vi "Ascenseur_Main.vi"() -> ()   [LabVIEW 2026]
panel:
  in  "Descente":bool
  in  "Montée":bool
  out "Vitesse Moteur":dbl
  out "Vitesse sauvegarder":dbl
  in  "Poids Max":dbl
  in  "Vitesse Max":dbl(slide) scale=0.0..10.0
  in  "Alarme":bool
  out "Poids cabine":dbl
  in  "baud rate (9600)":u32=9600
  in  "VISA resource name":refnum<visa-resource-name>
  out "Table Control":string[][](table)
  out "LCD":string
  out "Trames envoyés":string
  out "Trames Recues":string
  out "Dernier étage":dbl
  out "Trajets total":dbl
  out "Statut de connexion":string
  out "Connexion":bool
  out "Capteur IR":bool
  out "EEPROM prête":bool
  out "Cabine en mvt":bool
  out "Mode Manu":bool
  out "Mode Auto":bool
  out "Arrêt urgence":bool
  out "Alarme":bool
  out "Surcharge":bool
  out "Porte Ouverte":bool
  out "Connexion Active":bool
  out "Graphique 2 Poids en fonction du temps":dbl[](graph)
  out "Graphique 1 Position en fonction du temps":dbl[](graph)
  out "Nb trajet":dbl
  out "Direction":string
  out "Etage Actuel":dbl
  in  "Clear TX":bool
  in  "Clear RX":bool
  in  "RAFRAICHIR EEPROM":bool
  in  "ENVOYER CONFIG":bool
  in  "MANU":bool
  in  "AUTO":bool
  in  "Sauvegarder":bool
  in  "Clear":bool
  in  "Stop":bool
  in  "Start":bool
  in  "Déconnecter":bool
  in  "Connecter":bool
  in  "Reset Alarme":bool
  in  "Acquitement":bool
  in  "Arrêt urgence":bool
  in  "Fermeture Porte":bool
  in  "Ouverture Porte":bool
  in  "Etage 2":bool
  in  "Etage  3":bool
  in  "Etage 0":bool
  in  "Etage 1":bool
  # "Projet final du 2ème quadrimestre Système de controle d'ascenseur"
  # "Classe : 2AU"
  # "EL YAZAMI Yassine"
  # "TABICH Mohamed"
  # "Année académique : 2025-2026"
  # "Mode"
  # "Commandes"
  # "ETAT"
  # "INDICATEUR"
  # "Graphiques déroulants"
  # "Appel d'étage"
  # "CONFIG SEUILS"
  # "LCD"
  # "Données EEPROM"
  # "Historique des trajets"
  # "Mode Manuel"
  # "LOG COMMUNICATION"
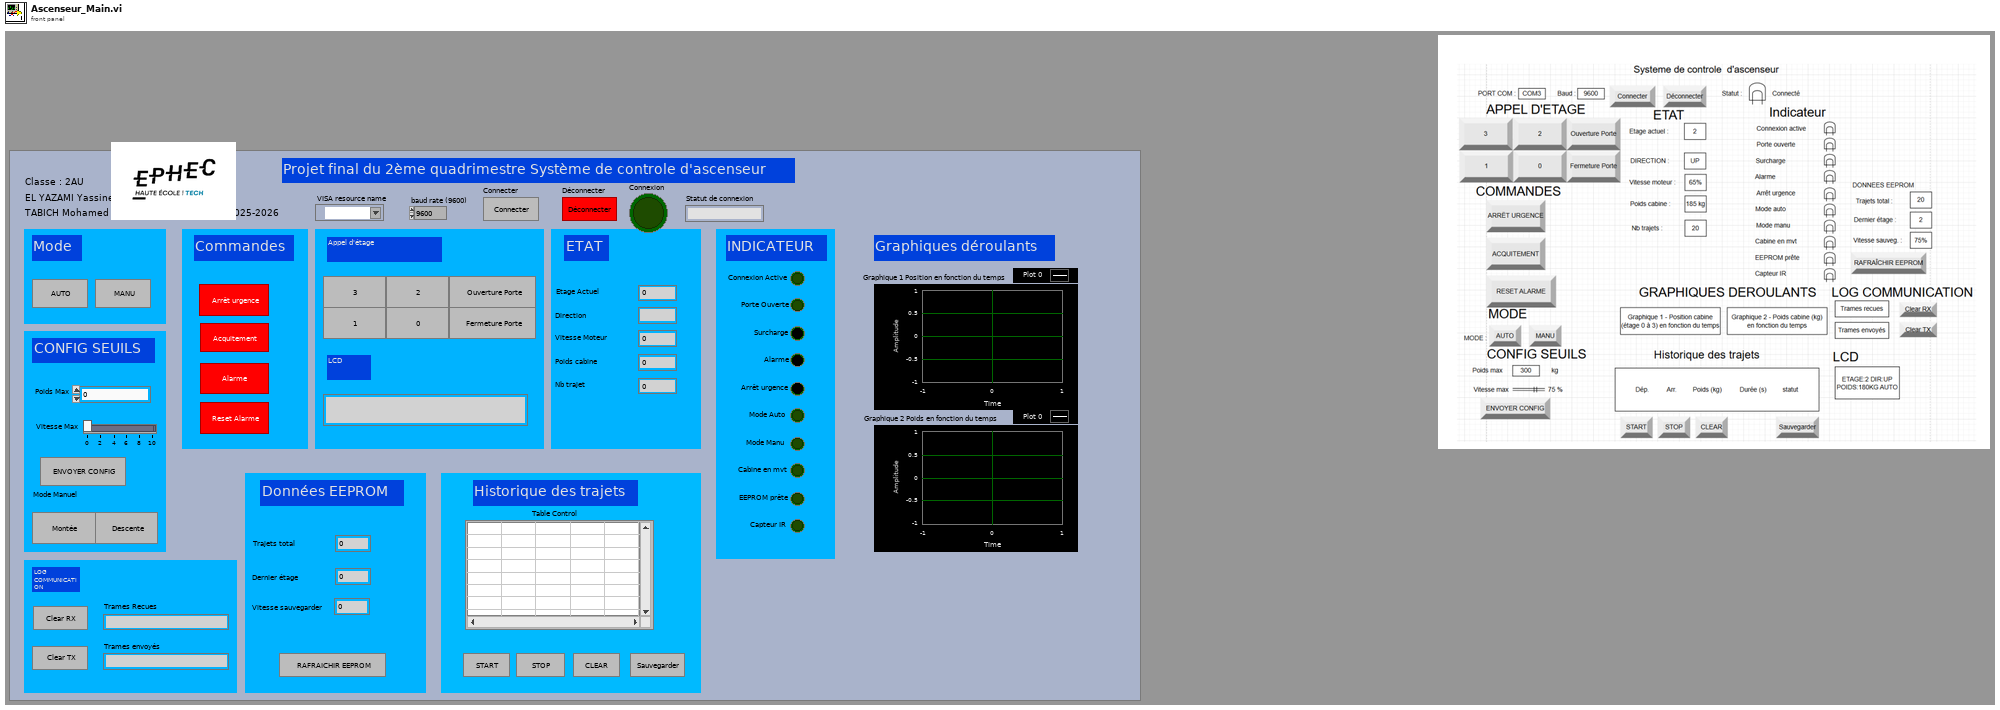
[diagram p1: front panel]
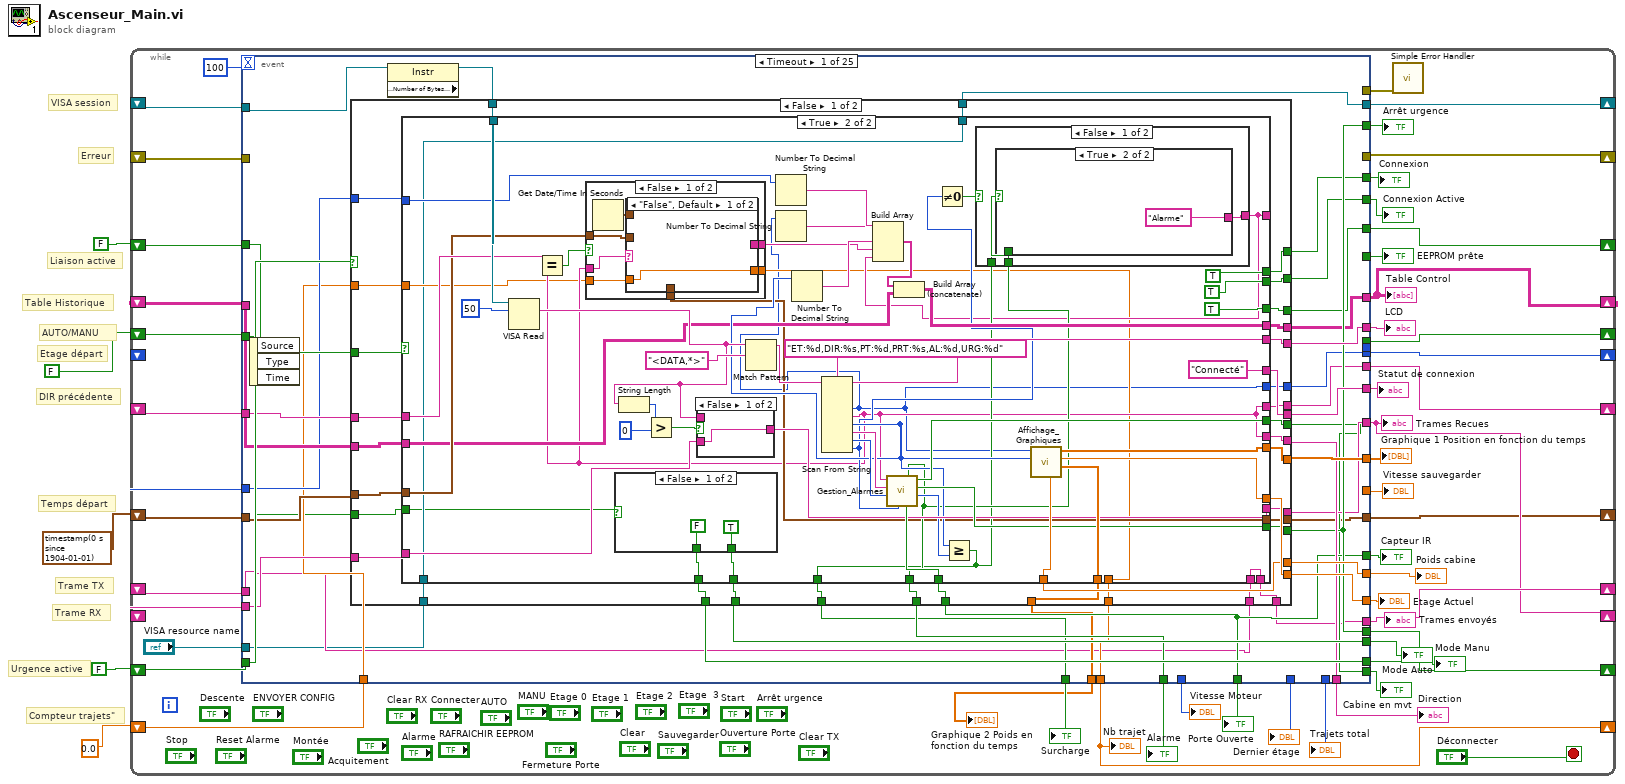
[diagram p0: block diagram]
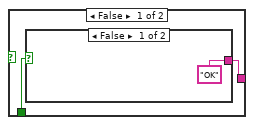
[diagram p3: hidden frame]
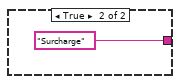
[diagram p4: hidden frame]
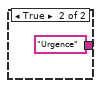
[diagram p5: hidden frame]
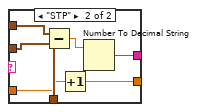
[diagram p6: hidden frame]
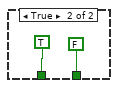
[diagram p9: hidden frame]
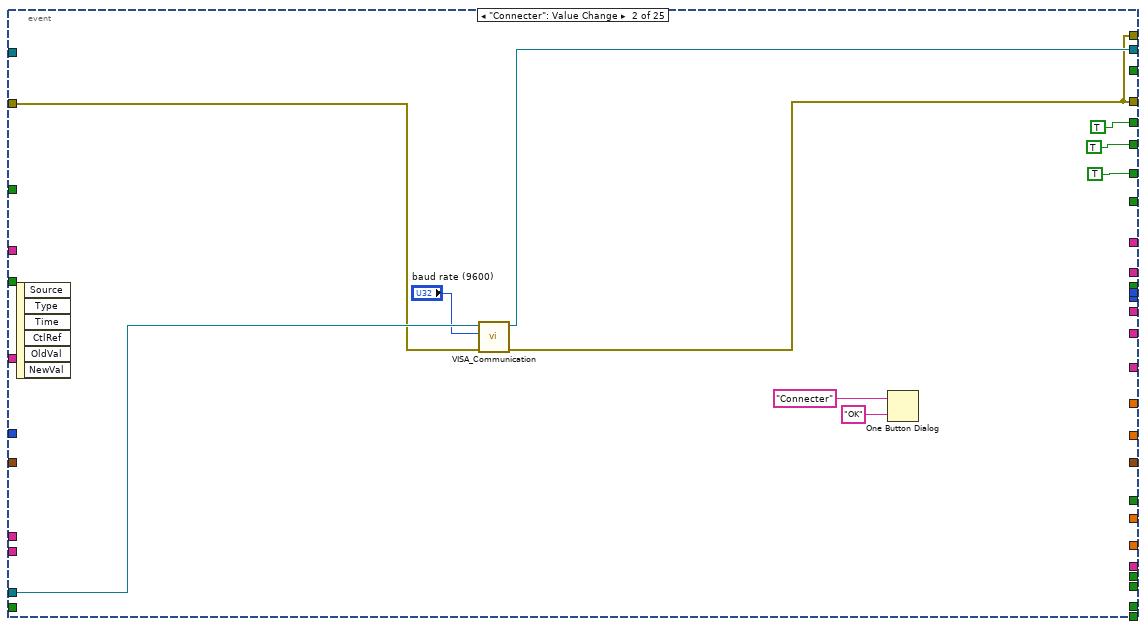
[diagram p11: hidden frame]
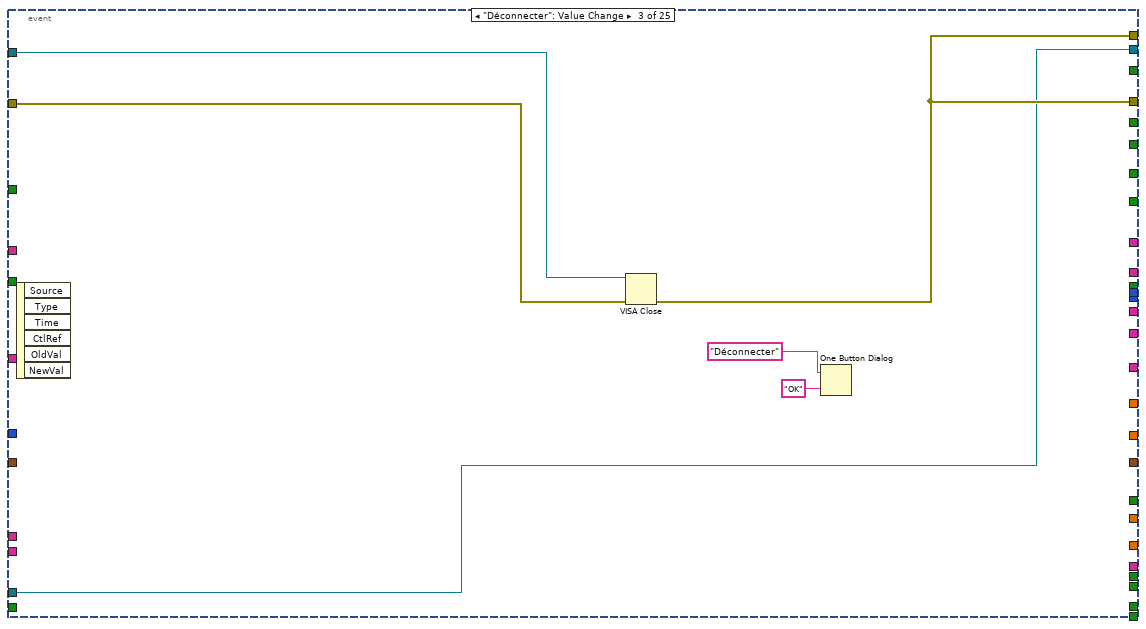
[diagram p12: hidden frame]
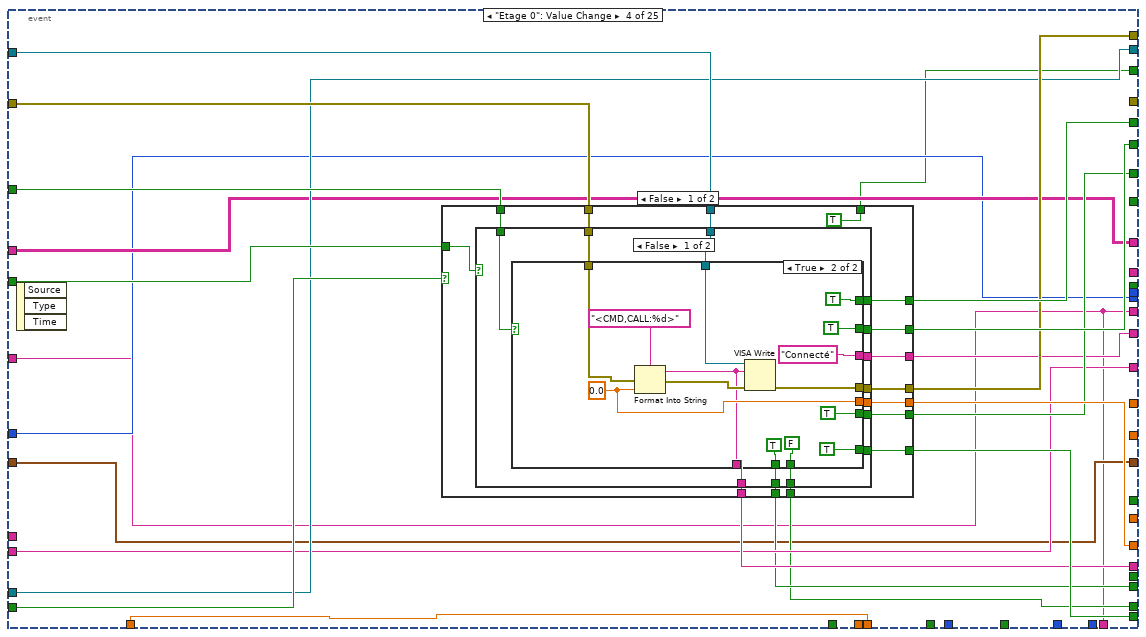
[diagram p13: hidden frame]
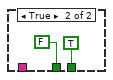
[diagram p15: hidden frame]
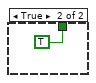
[diagram p16: hidden frame]
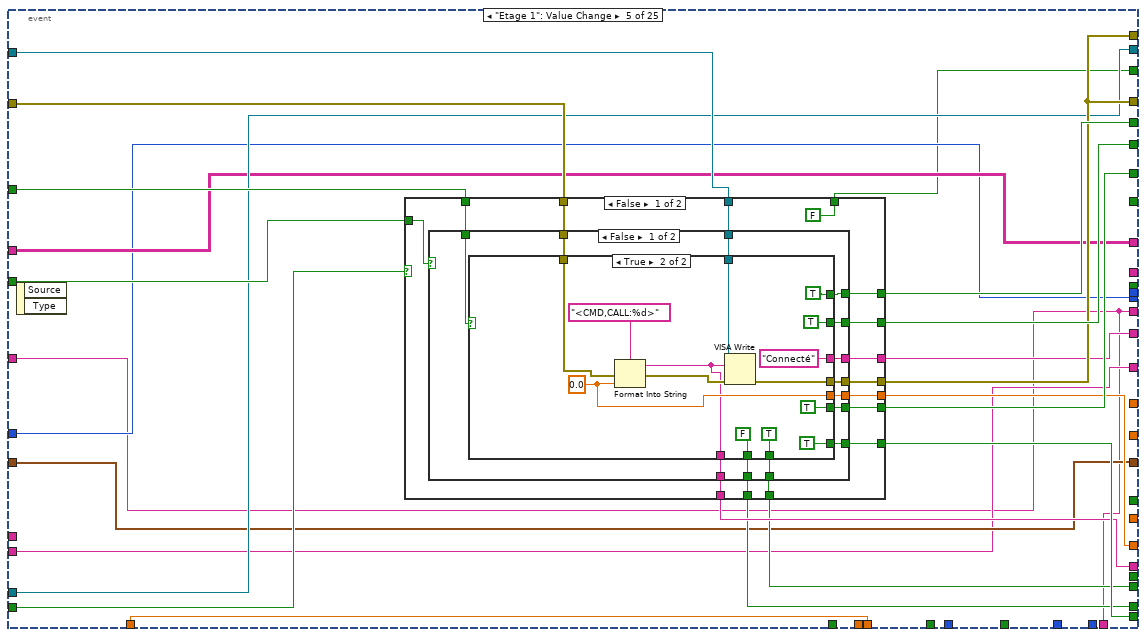
[diagram p17: hidden frame]
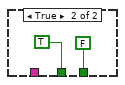
[diagram p19: hidden frame]
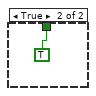
[diagram p20: hidden frame]
diagram:
  # "Compteur trajets\""
  # "Temps départ"
  # "Etage départ"
  # "Table Historique"
  # "DIR précédente"
  # "Trame RX"
  # "Urgence active"
  # "Trame TX"
  # "Erreur"
  # "VISA session"
  # "Liaison active"
  # "AUTO/MANU"
  n1 = while {
    shift-right: [w53] -> _
    shift-left: _ -> [w46]
    shift-right: [w52] -> _
    shift-left: _ -> [w50]
    shift-right: [w48] -> _
    shift-left: FALSE ("Enable Termination\nChar (T)") -> [w49]
    shift-right: [w29] -> _
    shift-left: FALSE ("Mode Auto") -> [w30]
    shift-right: [w28] -> _
    shift-left: _ -> [w45]
    shift-right: [w23] -> _
    shift-left: _ -> [w24]
    shift-right: [w32] -> _
    shift-left: FALSE ("Enable Termination\nChar (T)") -> [w31]
    shift-right: [w17] -> _
    shift-left: _ -> [w18]
    shift-right: [w10] -> _
    shift-left: _ -> [w16]
    shift-right: [w12] -> _
    shift-left: _ -> [w14]
    shift-right: [w11] -> _
    shift-left: timestamp(0 s since 1904-01-01) ("y") -> [w15]
    shift-right: [w7] -> _
    shift-left: 0.0 ("Nb trajet") -> [w9]
    stop <- "Déconnecter" stop-if-true
    n2 = event shown="[0] Timeout" {
      selector: _ -> [_ _ _ _ _ _ _ _ _ _ _ _ _ _ _ _ _ _ _ _ _ _ _ _ _]
      dyn-events: _ -> [_ _ _ _ _ _ _ _ _ _ _ _ _ _ _ _ _ _ _ _ _ _ _ _ _]
      timeout: 100 -> [_ _ _ _ _ _ _ _ _ _ _ _ _ _ _ _ _ _ _ _ _ _ _ _ _]
      tunnel: "VISA resource name" -> [w58 w221 w224 w239 w307 w377 w444 w513 w541 w588 w614 w647 w683 w734 w772 w835 w895 w953 w1006 w1059 w1083 w1115 w1137 w1148 w1175]
      tunnel: [w57 w219 w224 w239 w307 w377 w444 w513 w541 w588 w614 w647 w683 w734 w772 w835 w895 w953 w1006 w1059 w1083 w1115 w1137 w1148 w1175] -> w53
      tunnel: [_ w218 w226 _ w311 w370 w445 w515 w542 w580 w611 w645 w687 w736 w779 w836 w887 w952 w1005 w1056 w1080 w1113 w1134 w1157 w1177] -> w52
      tunnel: [_ w218 w226 w241 w311 w370 w445 w515 w542 w580 w611 w645 w687 w736 w779 w836 w887 w952 w1005 w1056 w1080 w1113 w1134 w1157 w1177] -> w51
      tunnel: w50 -> [_ w217 w225 w246 w309 w386 w439 w516 w544 w589 w618 w649 w693 w735 w782 w846 w897 w951 w1004 w1057 w1081 w1114 w1134 w1158 w1178]
      tunnel: w49 -> [w91 _ _ w249 w316 w380 w450 w511 w539 w585 w615 w646 w695 w739 w775 w834 w900 w955 w1009 w1055 w1076 w1107 w1122 w1155 w1179]
      tunnel: [w72 TRUE ("Enable Termination\nChar (T)") _ w243 w313 w382 w452 w506 w532 w581 w605 w637 w684 w729 w776 w840 w891 _ w1001 w1051 w1077 w1108 w1132 w1159 w1181] -> w48
      tunnel: [w74 TRUE ("Connexion") _ w250 w315 w385 w454 w508 w534 w583 w607 w639 w686 w731 w778 w842 w896 w946 w1003 w1053 w1079 w1110 w1133 w1160 w1183] -> w47
      tunnel: w46 -> [w93 _ w227 w240 w310 w381 w447 w517 w545 w590 w619 w650 w694 w737 w780 w847 w901 w954 w1010 w1058 w1082 _ _ _ _]
      tunnel: w45 -> [w68 _ _ w233 w302 w368 w435 w503 w540 w576 w608 w635 w679 w721 w767 w829 w881 w943 w994 w1048 w1068 _ w1136 w1151 w1172]
      tunnel: [w69 _ _ w233 w302 w368 w435 w503 w543 w576 w608 w635 w679 w721 w767 w829 w881 w943 w994 w1048 w1068 w1112 w1135 w1151 w1172] -> w28
      tunnel: [w73 TRUE ("Connexion Active") _ w244 w314 w384 w453 w507 w533 w582 w606 w638 w685 w730 w777 w841 w892 w949 w1002 w1052 w1078 w1109 w1131 w1156 w1182] -> w44
      tunnel: [w78 _ _ w236 w299 w371 w438 w504 w529 w577 w610 w634 w682 w725 w768 w833 w884 w941 w995 w1050 w1072 w1106 w1126 w1161 w1174] -> w17
      tunnel: [w59 _ _ w237 w305 w375 w442 w512 w536 w587 w616 w640 w692 w726 w769 w837 w888 w945 w998 w1054 w1073 w1105 w1127 w1149 w1180] -> w23
      tunnel: [w88 _ _ w238 w306 w376 w443 w510 w528 w586 w617 w643 w691 w733 w781 w843 w894 w948 w997 w1044 w1074 w1111 w1130 w1154 w1176] -> w43
      tunnel: [w86 _ _ w245 w308 w383 w446 _ _ _ _ _ _ _ _ _ _ _ _ _ _ _ _ _ _] -> w25
      tunnel: [w77 _ _ _ _ _ _ _ _ _ _ _ _ _ _ w839 w889 _ _ _ _ _ _ _ _] -> w42
      tunnel: [w89 _ _ w234 w303 w373 w440 _ _ _ _ _ w689 w727 _ _ w890 w944 w999 _ _ _ _ _ _] -> w41
      tunnel: [w90 _ _ w235 w304 w374 w441 _ _ _ _ _ w690 w728 _ _ _ _ _ _ _ _ _ _ _] -> w40
      tunnel: [w76 _ _ w242 w312 w372 w451 _ _ _ _ _ _ _ _ w838 _ w947 w1000 _ _ _ _ _ _] -> w39
      tunnel: [w80 _ _ w228 w296 w369 w432 w509 w535 w573 w609 _ _ _ _ _ _ _ _ _ _ _ _ _ _] -> w38
      tunnel: [w77 _ _ _ _ _ _ _ _ _ _ _ _ _ _ _ w893 _ _ _ _ _ _ _ _] -> w37
      tunnel: [w82 _ _ _ _ _ _ _ _ w584 w612 _ _ _ _ _ _ _ _ _ _ _ _ _ _] -> w36
      tunnel: [_ _ _ _ _ _ _ _ _ _ _ w642 _ _ _ _ _ _ _ _ _ _ _ _ _] -> w8
      tunnel: [_ _ _ _ _ _ _ _ _ _ _ w648 _ _ _ _ _ _ _ _ _ _ _ _ _] -> w35
      tunnel: [_ _ _ _ _ _ _ _ _ _ _ w644 _ _ w770 _ _ w950 _ _ _ _ _ _ _] -> w34
      tunnel: [w75 _ _ _ _ _ _ _ _ _ w613 _ _ _ _ _ _ _ _ _ _ _ _ _ _] -> w33
      tunnel: [w80 _ _ _ _ _ _ TRUE ("Enable Termination\nChar (T)") w537 _ _ _ _ _ _ _ _ _ _ _ _ _ w1123 w1152 w1173] -> w32
      tunnel: w31 -> [w92 _ _ w247 w318 w378 w448 _ w538 _ _ _ w696 w738 w774 w844 w898 w957 w1007 _ w1075 _ w1123 w1152 w1173]
      tunnel: w30 -> [w56 _ _ w248 w317 w379 w449 _ _ _ _ _ _ _ w773 w845 w899 w956 w1008 _ _ _ _ w1153 _]
      tunnel: [_ _ _ _ _ _ _ _ _ _ _ _ w688 w732 _ _ _ _ _ _ _ _ _ w1153 _] -> w29
      tunnel: [_ _ _ _ _ _ _ _ _ _ _ _ _ _ w771 _ _ _ _ _ _ _ _ _ _] -> w27
      tunnel: [_ _ _ _ _ _ _ _ _ _ _ w641 _ _ _ _ _ _ _ _ _ _ _ _ _] -> w26
      tunnel: w24 -> [w60 _ _ _ _ _ _ _ _ _ _ _ _ _ _ _ _ _ _ _ _ w1105 w1127 w1149 _]
      tunnel: [w87 _ _ _ _ _ _ _ _ _ _ _ _ _ _ _ _ _ _ _ _ _ _ _ _] -> w22
      tunnel: [w85 _ _ _ _ _ _ _ _ _ _ _ _ _ _ _ _ _ _ _ _ _ _ _ _] -> w21
      tunnel: [w84 _ _ _ _ _ _ _ _ _ _ _ _ _ _ _ _ _ _ _ _ _ _ _ _] -> w20
      tunnel: [w83 _ _ w229 w297 w364 w433 _ _ w574 w601 _ _ _ _ _ _ w939 w991 w1044 _ _ w1124 _ _] -> w19
      tunnel: w18 -> [w79 _ _ w236 w299 w371 w438 w504 w529 w577 w610 w634 w682 w725 w768 w833 w884 w941 w995 w1050 w1072 w1106 w1126 _ w1174]
      tunnel: w16 -> [w71 _ _ w229 w297 w364 w433 w505 w530 w574 w601 w636 w680 w723 w766 w828 w885 w939 w991 w1049 w1069 w1103 w1124 w1150 w1170]
      tunnel: w15 -> [w70 _ _ w231 w300 w366 w436 w500 _ w578 w603 w631 w678 w722 w765 w831 w882 w938 w992 w1045 w1071 w1102 w1129 w1146 w1171]
      tunnel: w14 -> [w67 _ _ w232 w301 w367 w434 w501 w527 w579 w604 w632 w681 w720 w763 w830 w886 w942 w993 w1046 w1070 w1104 w1125 w1147 w1168]
      tunnel: [w66 _ _ _ _ _ _ _ _ _ _ _ _ _ _ _ _ _ _ _ _ _ _ _ _] -> w13
      tunnel: [w65 _ _ w232 w301 w367 w434 w501 w527 w579 w604 w632 w681 w720 w763 w830 w886 w942 w993 w1046 w1070 w1104 w1125 w1147 _] -> w12
      tunnel: [w64 _ _ w231 w300 w366 w436 w500 _ w578 w603 w631 w678 w722 w765 w831 w882 w938 w992 w1045 w1071 w1102 w1129 w1146 w1171] -> w11
      tunnel: [w63 _ _ w229 w297 w364 w433 w505 w530 w574 w601 w636 w680 w723 w766 w828 w885 w939 w991 w1049 w1069 w1103 w1124 w1150 w1170] -> w10
      tunnel: w9 -> [w62 _ _ w230 w298 w365 w437 w502 w531 w575 w602 w633 w677 w724 w764 w832 w883 w940 w996 w1047 _ w1101 w1128 w1145 w1169]
      tunnel: [w61 _ _ w230 w298 w365 w437 w502 w531 w575 w602 w633 w677 w724 w764 w832 w883 w940 w996 w1047 _ w1101 w1128 w1145 w1169] -> w7
      tunnel: [_ _ _ _ _ _ _ _ _ _ _ _ _ _ _ _ _ _ _ _ _ _ _ _ w1168] -> _
      event Timeout {
        n3 = event-data() -> ()  [unwired: 1 in, 3 out]
        n4 = property class="Instr" props=["Serial Settings:Number of Bytes at Serial Port"](reference=w93) -> (reference out=w81:refnum<visa-resource-name>)  [unwired: 1 in, 2 out]
        n5 = case shown="False" w92 {
          tunnel: w91 -> [w129 _]
          tunnel: [w128 _] -> w90
          tunnel: [w127 _] -> w89
          tunnel: [w126 _] -> w88
          tunnel: [w125 _] -> w87
          tunnel: [w124 _] -> w86
          tunnel: [w123 _] -> w85
          tunnel: [w122 _] -> w66
          tunnel: [w121 _] -> w84
          tunnel: [w120 _] -> w83
          tunnel: [w119 _] -> w82
          tunnel: [w118 _] -> w77
          tunnel: w81 -> [w117 _]
          tunnel: [w116 _] -> w80
          tunnel: w79 -> [w115 _]
          tunnel: [w114 _] -> w78
          tunnel: [w113 _] -> w76
          tunnel: [w112 _] -> w75
          tunnel: [w111 _] -> w74
          tunnel: [w110 _] -> w73
          tunnel: [w109 _] -> w72
          tunnel: w71 -> [w108 _]
          tunnel: w70 -> [w107 _]
          tunnel: [w106 _] -> w69
          tunnel: w68 -> [w105 _]
          tunnel: w67 -> [w104 _]
          tunnel: [w103 _] -> w65
          tunnel: [w102 _] -> w64
          tunnel: [w101 _] -> w63
          tunnel: w62 -> [w100 _]
          tunnel: [w99 _] -> w61
          tunnel: w60 -> [w98 _]
          tunnel: [w97 _] -> w59
          tunnel: w58 -> [w96 _]
          tunnel: [w95 _] -> w57
          tunnel: w56 -> [w94 _]
          frame False {
            n6 = case shown="True" w129 {
              tunnel: [_ w136] -> w120
              tunnel: [_ w177] -> w118
              tunnel: [_ w140] -> w119
              tunnel: [_ w175] -> w121
              tunnel: [_ w174] -> w125
              tunnel: [_ w173] -> w124
              tunnel: [_ w172] -> w123
              tunnel: [_ w171] -> w122
              tunnel: [_ "Connecté" ("Statut de connexion")] -> w126
              tunnel: [_ w169] -> w128
              tunnel: [_ w168] -> w127
              tunnel: w117 -> [_ w167]
              tunnel: [_ w166] -> w116
              tunnel: w115 -> [_ w160]
              tunnel: [_ w161] -> w114
              tunnel: [_ w159] -> w113
              tunnel: [_ w139] -> w112
              tunnel: [_ TRUE ("Connexion")] -> w111
              tunnel: [_ TRUE ("Connexion Active")] -> w110
              tunnel: [_ TRUE ("Enable Termination\nChar (T)")] -> w109
              tunnel: w108 -> [_ w153]
              tunnel: w107 -> [_ w152]
              tunnel: [_ w151] -> w106
              tunnel: w105 -> [_ w144]
              tunnel: w104 -> [_ w150]
              tunnel: [_ w138] -> _
              tunnel: [_ w130] -> w103
              tunnel: [_ w137] -> w102
              tunnel: [_ w136] -> w101
              tunnel: w100 -> [_ w135]
              tunnel: [_ w134] -> w99
              tunnel: w98 -> [_ w133]
              tunnel: [_ w133] -> w97
              tunnel: [_ w132] -> w95
              tunnel: w96 -> [_ w132]
              tunnel: w94 -> [_ w131]
              frame False {
              }
              frame True {
                n7 = VISA Read(VISA resource name=w167, byte count=u32 50) -> (read buffer=w162:string)  [unwired: 1 in, 3 out]
                n8 = case shown="False" w131 {
                  tunnel: [TRUE ("Mode Auto") FALSE ("Mode Auto")] -> w169
                  tunnel: [FALSE ("Mode Manu") TRUE ("Mode Manu")] -> w168
                  frame False {
                  }
                  frame True {
                  }
                }
                n9 = String Length(string=w162) -> (length=w164:i32)
                n10 = Greater?(x=w164, y=0 ("length")) -> (0:w163:bool)
                n11 = case shown="False" w163 {
                  tunnel: [w206 w207] -> w161
                  tunnel: w162 -> [_ w207]
                  tunnel: w160 -> [w206 _]
                  frame False {
                  }
                  frame True {
                  }
                }
                n12 = Match Pattern(string=w162, regular expression="<DATA,*>") -> (after substring=w180:string)  [unwired: 1 in, 3 out]
                n13 = Number To Decimal String(number=w150) -> (decimal integer string=w148:string)  [unwired: 1 in]
                n14 = Scan From String(format string="ET:%d,DIR:%s,PT:%d,PRT:%s,AL:%d,URG:%d", input string=w180) -> (remaining string=w175:string, output 1=w130:i32, output 2=w136:string, output 3=w149:i32, output 4=w178:string, output 5=w176:i32, output 6=w141:i32)  [unwired: 8 in, 2 out]
                n15 = Equal?(x=w153, y=w136) -> (x = y?=w154:bool)
                n16 = case shown="False" w154 {
                  tunnel: w136 -> [w198 _]
                  tunnel: w152 -> [w196 _]
                  tunnel: [w195 _] -> w145
                  tunnel: [w194 _] -> w137
                  tunnel: w135 -> [w193 _]
                  tunnel: [w192 _] -> w134
                  frame False {
                    n17 = Get Date/Time In Seconds() -> (seconds since 1Jan1904=w197:timestamp)
                    n18 = case shown="\"False\", Default" w198 {
                      tunnel: w197 -> [_ w205]
                      tunnel: w196 -> [_ w202]
                      tunnel: [_ w203] -> w195
                      tunnel: [_ w202] -> w194
                      tunnel: w193 -> [w199 w201]
                      tunnel: [w199 w200] -> w192
                      frame "False", Default {
                      }
                      frame "STP" {
                        n19 = Subtract(x=w205, y=w202) -> (x-y=w204:dbl)
                        n20 = Increment(x=w201) -> (x+1=w200:dbl)
                        n21 = Number To Decimal String(number=w204) -> (decimal integer string=w203:string)  [unwired: 1 in]
                      }
                    }
                  }
                  frame True {
                  }
                }
                n22 = Number To Decimal String(number=w130) -> (decimal integer string=w147:string)  [unwired: 1 in]
                n23 = Number To Decimal String(number=w149) -> (decimal integer string=w146:string)  [unwired: 1 in]
                n24 = call "Gestion_Alarmes.vi"("Numeric"=w141, "Numeric 2"=w176, "String 2"=w178, "String"=w136) -> ("y"=w158:i32, "Boolean 3"=w166:bool, "Boolean 2"=w159:bool, "Boolean 4"=w177:bool, "Boolean"=w140:bool)  [unwired: 3 in]
                n25 = Not Equal To 0?(x=w141) -> (x != 0?=w142:bool)
                n26 = Greater Or Equal?(x=w149, y=w158) -> (x >= y?=w139:bool)
                n27 = case shown="False" w142 {
                  tunnel: w140 -> [w185 _]
                  tunnel: w139 -> [w184 _]
                  tunnel: [w183 "Urgence"] -> w138
                  frame False {
                    n28 = case shown="True" w185 {
                      tunnel: w184 -> [w187 _]
                      tunnel: [w186 "Alarme"] -> w183
                      frame False {
                        n29 = case shown="False" w187 {
                          tunnel: ["OK" "Surcharge"] -> w186
                          frame False {
                          }
                          frame True {
                          }
                        }
                      }
                      frame True {
                      }
                    }
                  }
                  frame True {
                  }
                }
                n30 = Build Array(w148, w147, w146, w145, w138) -> (w143:string[])
                n31 = Build Array (concatenate)(w143, w144) -> (w151:string[][])
                n32 = call "Affichage_Graphiques.vi"("Poids"=w149, "Position"=w130) -> ("Graphique 2 Poids en fonction du temps"=w171:dbl[], "Etage Actuel"=w173:dbl, "Graphique 1 Position en fonction du temps"=w174:dbl[], "Poids cabine"=w172:dbl)  [unwired: 6 in]
              }
            }
          }
          frame True {
          }
        }
      }
      event "Connecter": Value Change {
        n33 = event-data() -> ()  [unwired: 1 in, 6 out]
        n34 = call "VISA_Communication.vi"("error in (no error)"=w217, "baud rate (9600)"="baud rate (9600)", "VISA Refnum in"=w221) -> ("error out"=w218:errorcluster, "VISA Refnum out"=w219:refnum<visa-resource-name>)  [unwired: 7 in]
        n35 = One Button Dialog(message="Connecter", button name ("OK")="OK") -> ()  [unwired: 1 out]
      }
      event "Déconnecter": Value Change {
        n36 = event-data() -> ()  [unwired: 1 in, 6 out]
        n37 = VISA Close(VISA resource name=w227, error in (no error)=w225) -> (error out=w226:errorcluster)
        n38 = One Button Dialog(message="Déconnecter", button name ("OK")="OK") -> ()  [unwired: 1 out]
      }
      event "Etage 0": Value Change {
        n39 = event-data() -> ()  [unwired: 1 in, 3 out]
        n40 = case shown="False" w247 {
          tunnel: [w265 _] -> w250
          tunnel: w249 -> [w264 _]
          tunnel: w248 -> [w263 _]
          tunnel: w246 -> [w262 _]
          tunnel: [w261 _] -> w245
          tunnel: [w260 _] -> w244
          tunnel: [w259 _] -> w243
          tunnel: [w258 _] -> w242
          tunnel: [w257 _] -> w241
          tunnel: w240 -> [w256 _]
          tunnel: [w255 _] -> w238
          tunnel: [w254 _] -> w237
          tunnel: [w253 _] -> w235
          tunnel: [w252 _] -> w234
          tunnel: [TRUE ("Connexion") TRUE ("Connexion")] -> w228
          frame False {
            n41 = case shown="False" w263 {
              tunnel: [w278 _] -> w265
              tunnel: w264 -> [w277 _]
              tunnel: w262 -> [w276 _]
              tunnel: [w275 _] -> w261
              tunnel: [w274 _] -> w260
              tunnel: [w273 _] -> w259
              tunnel: [w272 _] -> w258
              tunnel: [w271 _] -> w257
              tunnel: w256 -> [w270 _]
              tunnel: [w269 _] -> w255
              tunnel: [w268 _] -> w254
              tunnel: [w267 FALSE ("Mode Auto")] -> w253
              tunnel: [w266 TRUE ("Mode Manu")] -> w252
              frame False {
                n42 = case shown="True" w277 {
                  tunnel: [_ w291] -> w271
                  tunnel: [_ TRUE ("Enable Termination\nChar (T)")] -> w273
                  tunnel: [_ TRUE ("Connexion")] -> w278
                  tunnel: [_ w287] -> w275
                  tunnel: [_ TRUE ("Cabine en mvt")] -> w272
                  tunnel: w276 -> [_ w285]
                  tunnel: [_ TRUE ("Connexion Active")] -> w274
                  tunnel: w270 -> [_ w283]
                  tunnel: [_ "Connecté" ("Statut de connexion")] -> w269
                  tunnel: [_ w281] -> w268
                  tunnel: [_ TRUE ("Mode Auto")] -> w267
                  tunnel: [_ FALSE ("Mode Manu")] -> w266
                  frame False {
                  }
                  frame True {
                    w287 = 0.0 ("input 1")
                    n43 = Format Into String(format string="<CMD,CALL:%d>", error in=w285, w287) -> (resulting string=w281:string, error out=w288:errorcluster)  [unwired: 1 in]
                    n44 = VISA Write(VISA resource name=w283, write buffer=w281, error in (no error)=w288) -> (error out=w291:errorcluster)  [unwired: 2 out]
                  }
                }
              }
              frame True {
              }
            }
          }
          frame True {
          }
        }
      }
      event "Etage 1": Value Change {
        n45 = event-data() -> ()  [unwired: 1 in, 2 out]
        n46 = case shown="False" w318 {
          tunnel: [w333 _] -> w315
          tunnel: [w332 _] -> w308
          tunnel: [w331 _] -> w314
          tunnel: [w330 _] -> w313
          tunnel: [w329 _] -> w312
          tunnel: w317 -> [w328 _]
          tunnel: w316 -> [w327 _]
          tunnel: [w326 _] -> w311
          tunnel: w310 -> [w325 _]
          tunnel: w309 -> [w324 _]
          tunnel: [w323 _] -> w306
          tunnel: [w322 _] -> w305
          tunnel: [w321 _] -> w304
          tunnel: [w320 _] -> w303
          tunnel: [FALSE ("Connexion") TRUE ("Connexion")] -> w296
          frame False {
            n47 = case shown="False" w328 {
              tunnel: [w346 _] -> w333
              tunnel: [w345 _] -> w332
              tunnel: [w344 _] -> w331
              tunnel: [w343 _] -> w330
              tunnel: [w342 _] -> w329
              tunnel: w327 -> [w341 _]
              tunnel: [w340 _] -> w326
              tunnel: w325 -> [w339 _]
              tunnel: w324 -> [w338 _]
              tunnel: [w337 _] -> w323
              tunnel: [w336 _] -> w322
              tunnel: [w335 FALSE ("Mode Auto")] -> w321
              tunnel: [w334 TRUE ("Mode Manu")] -> w320
              frame False {
                n48 = case shown="True" w341 {
                  tunnel: [_ w359] -> w340
                  tunnel: [_ TRUE ("Enable Termination\nChar (T)")] -> w343
                  tunnel: [_ TRUE ("Connexion")] -> w346
                  tunnel: [_ w355] -> w345
                  tunnel: [_ TRUE ("Cabine en mvt")] -> w342
                  tunnel: [_ TRUE ("Connexion Active")] -> w344
                  tunnel: w339 -> [_ w352]
                  tunnel: w338 -> [_ w351]
                  tunnel: [_ "Connecté" ("Statut de connexion")] -> w337
                  tunnel: [_ w349] -> w336
                  tunnel: [_ TRUE ("Mode Auto")] -> w335
                  tunnel: [_ FALSE ("Mode Manu")] -> w334
                  frame False {
                  }
                  frame True {
                    w355 = 0.0 ("input 1")
                    n49 = Format Into String(format string="<CMD,CALL:%d>", error in=w351, w355) -> (resulting string=w349:string, error out=w356:errorcluster)  [unwired: 1 in]
                    n50 = VISA Write(VISA resource name=w352, write buffer=w349, error in (no error)=w356) -> (error out=w359:errorcluster)  [unwired: 2 out]
                  }
                }
              }
              frame True {
              }
            }
          }
          frame True {
          }
        }
      }
      event "Etage 2": Value Change {
        n51 = event-data() -> ()  [unwired: 1 in, 3 out]
        n52 = case shown="False" w378 {
          tunnel: [w401 _] -> w385
          tunnel: [w400 _] -> w383
          tunnel: [w399 _] -> w384
          tunnel: [w398 _] -> w382
          tunnel: [w397 _] -> w372
          tunnel: [w396 _] -> w370
          tunnel: w386 -> [w395 _]
          tunnel: w381 -> [w394 _]
          tunnel: w380 -> [w393 _]
          tunnel: w379 -> [w392 _]
          tunnel: [w391 _] -> w376
          tunnel: [w390 _] -> w375
          tunnel: [w389 _] -> w374
          tunnel: [w388 _] -> w373
          tunnel: [FALSE ("Arrêt urgence") TRUE ("Arrêt urgence")] -> w369
          frame False {
            n53 = case shown="False" w392 {
              tunnel: [w414 _] -> w401
              tunnel: [w413 _] -> w400
              tunnel: [w412 _] -> w399
              tunnel: [w411 _] -> w398
              tunnel: [w410 _] -> w397
              tunnel: [w409 _] -> w396
              tunnel: w395 -> [w408 _]
              tunnel: w394 -> [w407 _]
              tunnel: w393 -> [w406 _]
              tunnel: [w405 _] -> w391
              tunnel: [w404 _] -> w390
              tunnel: [w403 FALSE ("Mode Auto")] -> w389
              tunnel: [w402 TRUE ("Mode Manu")] -> w388
              frame False {
                n54 = case shown="True" w406 {
                  tunnel: [_ w427] -> w409
                  tunnel: [_ TRUE ("Enable Termination\nChar (T)")] -> w411
                  tunnel: [_ TRUE ("Connexion")] -> w414
                  tunnel: [_ w423] -> w413
                  tunnel: [_ TRUE ("Cabine en mvt")] -> w410
                  tunnel: [_ TRUE ("Connexion Active")] -> w412
                  tunnel: w408 -> [_ w420]
                  tunnel: w407 -> [_ w419]
                  tunnel: [_ "Connecté" ("Statut de connexion")] -> w405
                  tunnel: [_ w417] -> w404
                  tunnel: [_ TRUE ("Mode Auto")] -> w403
                  tunnel: [_ FALSE ("Mode Manu")] -> w402
                  frame False {
                  }
                  frame True {
                    w423 = 0.0 ("input 1")
                    n55 = Format Into String(format string="<CMD,CALL:%d>", error in=w420, w423) -> (resulting string=w417:string, error out=w424:errorcluster)  [unwired: 1 in]
                    n56 = VISA Write(VISA resource name=w419, write buffer=w417, error in (no error)=w424) -> (error out=w427:errorcluster)  [unwired: 2 out]
                  }
                }
              }
              frame True {
              }
            }
          }
          frame True {
          }
        }
      }
      event "Etage  3": Value Change {
        n57 = event-data() -> ()  [unwired: 1 in, 3 out]
        n58 = case shown="False" w448 {
          tunnel: [w469 _] -> w454
          tunnel: [w468 _] -> w446
          tunnel: [w467 _] -> w453
          tunnel: [w466 _] -> w452
          tunnel: [w465 _] -> w451
          tunnel: [w464 _] -> w445
          tunnel: w450 -> [w463 _]
          tunnel: w449 -> [w462 _]
          tunnel: w447 -> [w461 _]
          tunnel: [w460 _] -> w443
          tunnel: [w459 _] -> w442
          tunnel: [w458 _] -> w441
          tunnel: [w457 _] -> w440
          tunnel: w439 -> [w456 _]
          tunnel: [FALSE ("Arrêt urgence") TRUE ("Arrêt urgence")] -> w432
          frame False {
            n59 = case shown="False" w462 {
              tunnel: [w482 _] -> w469
              tunnel: [w481 _] -> w468
              tunnel: [w480 _] -> w467
              tunnel: [w479 _] -> w466
              tunnel: [w478 _] -> w465
              tunnel: [w477 _] -> w464
              tunnel: w463 -> [w476 _]
              tunnel: w461 -> [w475 _]
              tunnel: [w474 _] -> w460
              tunnel: [w473 _] -> w459
              tunnel: [w472 FALSE ("Mode Auto")] -> w458
              tunnel: [w471 TRUE ("Mode Manu")] -> w457
              tunnel: w456 -> [w470 _]
              frame False {
                n60 = case shown="True" w476 {
                  tunnel: [_ w495] -> w477
                  tunnel: [_ TRUE ("Enable Termination\nChar (T)")] -> w479
                  tunnel: [_ TRUE ("Connexion")] -> w482
                  tunnel: [_ w491] -> w481
                  tunnel: [_ TRUE ("Cabine en mvt")] -> w478
                  tunnel: [_ TRUE ("Connexion Active")] -> w480
                  tunnel: w475 -> [_ w488]
                  tunnel: [_ "Connecté" ("Statut de connexion")] -> w474
                  tunnel: [_ w486] -> w473
                  tunnel: [_ TRUE ("Mode Auto")] -> w472
                  tunnel: [_ FALSE ("Mode Manu")] -> w471
                  tunnel: w470 -> [_ w483]
                  frame False {
                  }
                  frame True {
                    w491 = 0.0 ("input 1")
                    n61 = Format Into String(format string="<CMD,CALL:%d>", error in=w483, w491) -> (resulting string=w486:string, error out=w492:errorcluster)  [unwired: 1 in]
                    n62 = VISA Write(VISA resource name=w488, write buffer=w486, error in (no error)=w492) -> (error out=w495:errorcluster)  [unwired: 2 out]
                  }
                }
              }
              frame True {
              }
            }
          }
          frame True {
          }
        }
      }
      event "Arrêt urgence": Value Change {
        n63 = event-data() -> ()  [unwired: 1 in, 3 out]
        n64 = case shown="True" w511 {
          tunnel: w517 -> [_ w526]
          tunnel: w516 -> [_ w525]
          tunnel: [_ w524] -> w515
          tunnel: [_ w523] -> w512
          tunnel: [_ "URGENCE DÉCLENCHÉE" ("Statut de connexion")] -> w510
          tunnel: [_ TRUE ("Arrêt urgence")] -> w509
          tunnel: [_ TRUE ("Connexion")] -> w508
          tunnel: [_ TRUE ("Connexion Active")] -> w507
          tunnel: [_ TRUE ("Enable Termination\nChar (T)")] -> w506
          frame False {
          }
          frame True {
            w523 = "<CMD,STOP>"
            n65 = VISA Write(VISA resource name=w526, write buffer=w523, error in (no error)=w525) -> (error out=w524:errorcluster)  [unwired: 2 out]
          }
        }
      }
      event "Acquitement": Value Change {
        n66 = event-data() -> ()  [unwired: 1 in, 3 out]
        n67 = case shown="True" w538 {
          tunnel: w545 -> [_ w558]
          tunnel: w544 -> [_ w557]
          tunnel: [_ w556] -> w543
          tunnel: [_ w555] -> w542
          tunnel: w540 -> [_ w554]
          tunnel: w539 -> [_ w553]
          tunnel: [_ w552] -> w537
          tunnel: [_ w551] -> w536
          tunnel: [_ w550] -> w535
          tunnel: [_ w549] -> w534
          tunnel: [_ w548] -> w533
          tunnel: [_ w547] -> w532
          tunnel: [_ w546] -> w528
          frame False {
          }
          frame True {
            n68 = case shown="True" w553 {
              tunnel: w558 -> [_ w572]
              tunnel: w557 -> [_ w571]
              tunnel: [_ w568] -> w556
              tunnel: [_ w567] -> w555
              tunnel: w554 -> [_ w565]
              tunnel: [_ FALSE ("Enable Termination\nChar (T)")] -> w552
              tunnel: [_ w564] -> w551
              tunnel: [_ FALSE ("Arrêt urgence")] -> w550
              tunnel: [_ TRUE ("Connexion")] -> w549
              tunnel: [_ TRUE ("Connexion Active")] -> w548
              tunnel: [_ TRUE ("Enable Termination\nChar (T)")] -> w547
              tunnel: [_ "Système réinitialisé" ("Statut de connexion")] -> w546
              frame False {
              }
              frame True {
                w564 = "<CMD,ACK> "
                n69 = Build Array("TX: <CMD,ACK> " ("Statut de connexion")) -> (w569:string[])
                n70 = VISA Write(VISA resource name=w572, write buffer=w564, error in (no error)=w571) -> (error out=w567:errorcluster)  [unwired: 2 out]
                n71 = Build Array (concatenate)(w569, w565) -> (w568:string[][])
              }
            }
          }
        }
      }
      event "Alarme": Value Change {
        n72 = event-data() -> ()  [unwired: 1 in, 3 out]
        n73 = case shown="True" w585 {
          tunnel: w590 -> [_ w600]
          tunnel: w589 -> [_ w599]
          tunnel: [_ w596] -> w580
          tunnel: [_ w598] -> w587
          tunnel: [_ "Alarme déclenchée " ("Statut de connexion")] -> w586
          tunnel: [_ TRUE] -> w584
          tunnel: [_ TRUE ("Connexion")] -> w583
          tunnel: [_ TRUE ("Connexion Active")] -> w582
          tunnel: [_ TRUE ("Enable Termination\nChar (T)")] -> w581
          tunnel: [_ FALSE ("Arrêt urgence")] -> w573
          frame False {
          }
          frame True {
            w598 = "<CMD,AL:ON> "
            n74 = VISA Write(VISA resource name=w600, write buffer=w598, error in (no error)=w599) -> (error out=w596:errorcluster)  [unwired: 2 out]
          }
        }
      }
      event "Reset Alarme": Value Change {
        n75 = event-data() -> ()  [unwired: 1 in, 3 out]
        n76 = case shown="True" w615 {
          tunnel: w619 -> [_ w630]
          tunnel: w618 -> [_ w629]
          tunnel: [_ w628] -> w611
          tunnel: [_ "Alarmes réinitialisées " ("Statut de connexion")] -> w617
          tunnel: [_ w626] -> w616
          tunnel: [_ FALSE ("Surcharge")] -> w613
          tunnel: [_ FALSE] -> w612
          tunnel: [_ FALSE] -> w609
          tunnel: [_ TRUE ("Connexion")] -> w607
          tunnel: [_ TRUE ("Connexion Active")] -> w606
          tunnel: [_ TRUE ("Enable Termination\nChar (T)")] -> w605
          frame False {
          }
          frame True {
            w626 = "<CMD,RST:AL> "
            n77 = VISA Write(VISA resource name=w630, write buffer=w626, error in (no error)=w629) -> (error out=w628:errorcluster)  [unwired: 2 out]
          }
        }
      }
      event "RAFRAICHIR EEPROM": Value Change {
        n78 = event-data() -> ()  [unwired: 1 in, 3 out]
        n79 = case shown="True" w646 {
          tunnel: w650 -> [_ w675]
          tunnel: w649 -> [_ w674]
          tunnel: [_ w662] -> w642
          tunnel: [_ w665] -> w648
          tunnel: [_ w663] -> w645
          tunnel: [_ TRUE ("EEPROM prête")] -> w644
          tunnel: [_ "Connecté" ("Statut de connexion")] -> w643
          tunnel: [_ w657] -> w641
          tunnel: [_ w654] -> w640
          tunnel: [_ TRUE ("Connexion")] -> w639
          tunnel: [_ TRUE ("Connexion Active")] -> w638
          tunnel: [_ TRUE ("Enable Termination\nChar (T)")] -> w637
          frame False {
          }
          frame True {
            w654 = "<CMD,GET:EEP>" ("write buffer")
            n80 = VISA Write(VISA resource name=w675, write buffer=w654, error in (no error)=w674) -> (VISA resource name out=w670:refnum<visa-resource-name>, error out=w664:errorcluster)  [unwired: 1 out]
            n81 = Wait (ms)(milliseconds to wait=u32 500) -> ()  [unwired: 1 out]
            n82 = VISA Read(VISA resource name=w670, byte count=u32 128, error in (no error)=w664) -> (read buffer=w669:string, error out=w663:errorcluster)  [unwired: 2 out]
            n83 = Match Pattern(string=w669, regular expression="TRAJ:") -> (after substring=w667:string)  [unwired: 1 in, 3 out]
            n84 = Match Pattern(string=w667, regular expression="LAST:") -> (after substring=w656:string)  [unwired: 1 in, 3 out]
            n85 = Match Pattern(string=w656, regular expression="VITESSE") -> (before substring=w655:string)  [unwired: 1 in, 3 out]
            n86 = Scan From String(format string="%d", input string=w655) -> (output 1=w657:i32)  [unwired: 3 in, 3 out]
            n87 = Scan From String(format string="%d", input string=w667) -> (output 1=w662:i32)  [unwired: 3 in, 3 out]
            n88 = Scan From String(format string="%d", input string=w656) -> (output 1=w665:i32)  [unwired: 3 in, 3 out]
          }
        }
      }
      event "Mode Auto": Value Change {
        n89 = event-data() -> ()  [unwired: 1 in, 3 out]
        n90 = case shown="False" w696 {
          tunnel: w695 -> [w708 _]
          tunnel: [w707 _] -> w687
          tunnel: w694 -> [w706 _]
          tunnel: w693 -> [w705 _]
          tunnel: [w704 _] -> w692
          tunnel: [w703 _] -> w691
          tunnel: [w702 _] -> w690
          tunnel: [w701 _] -> w689
          tunnel: [w700 _] -> w688
          tunnel: [w699 _] -> w686
          tunnel: [w698 _] -> w685
          tunnel: [w697 _] -> w684
          frame False {
            n91 = case shown="True" w708 {
              tunnel: [_ w719] -> w707
              tunnel: w706 -> [_ w718]
              tunnel: w705 -> [_ w717]
              tunnel: [_ w716] -> w704
              tunnel: [_ "Connecté" ("Statut de connexion")] -> w703
              tunnel: [_ TRUE ("Mode Auto")] -> w702
              tunnel: [_ FALSE ("Mode Manu")] -> w701
              tunnel: [_ FALSE ("Mode Auto")] -> w700
              tunnel: [_ TRUE ("Connexion")] -> w699
              tunnel: [_ TRUE ("Connexion Active")] -> w698
              tunnel: [_ TRUE ("Enable Termination\nChar (T)")] -> w697
              frame False {
              }
              frame True {
                w716 = "<CMD,MODE:AUTO> " ("write buffer")
                n92 = VISA Write(VISA resource name=w718, write buffer=w716, error in (no error)=w717) -> (error out=w719:errorcluster)  [unwired: 2 out]
              }
            }
          }
          frame True {
          }
        }
      }
      event "Mode Manu": Value Change {
        n93 = event-data() -> ()  [unwired: 1 in, 3 out]
        n94 = case shown="False" w738 {
          tunnel: w739 -> [w751 _]
          tunnel: w737 -> [w750 _]
          tunnel: [w749 _] -> w736
          tunnel: w735 -> [w748 _]
          tunnel: [w747 _] -> w733
          tunnel: [w746 _] -> w732
          tunnel: [w745 _] -> w731
          tunnel: [w744 _] -> w730
          tunnel: [w743 _] -> w729
          tunnel: [w742 _] -> w728
          tunnel: [w741 _] -> w727
          tunnel: [w740 _] -> w726
          frame False {
            n95 = case shown="True" w751 {
              tunnel: w750 -> [_ w762]
              tunnel: [_ w761] -> w749
              tunnel: w748 -> [_ w760]
              tunnel: [_ "Connecté" ("Statut de connexion")] -> w747
              tunnel: [_ TRUE ("Mode Auto")] -> w746
              tunnel: [_ TRUE ("Connexion")] -> w745
              tunnel: [_ TRUE ("Connexion Active")] -> w744
              tunnel: [_ TRUE ("Enable Termination\nChar (T)")] -> w743
              tunnel: [_ FALSE ("Mode Auto")] -> w742
              tunnel: [_ TRUE ("Mode Manu")] -> w741
              tunnel: [_ w752] -> w740
              frame False {
              }
              frame True {
                w752 = "<CMD,MODE:MAN> " ("write buffer")
                n96 = VISA Write(VISA resource name=w762, write buffer=w752, error in (no error)=w760) -> (error out=w761:errorcluster)  [unwired: 2 out]
              }
            }
          }
          frame True {
          }
        }
      }
      event "ENVOYER CONFIG": Value Change {
        n97 = event-data() -> ()  [unwired: 1 in, 3 out]
        n98 = case shown="False" w774 {
          tunnel: w782 -> [w794 _]
          tunnel: [w793 _] -> w781
          tunnel: w780 -> [w792 _]
          tunnel: [w791 _] -> w779
          tunnel: [w790 _] -> w778
          tunnel: [w789 _] -> w777
          tunnel: [w788 _] -> w776
          tunnel: w775 -> [w787 _]
          tunnel: w773 -> [w786 _]
          tunnel: [w785 _] -> w771
          tunnel: [w784 _] -> w770
          tunnel: [w783 _] -> w769
          frame False {
            n99 = case shown="True" w786 {
              tunnel: w794 -> [_ w805]
              tunnel: [_ w804] -> w790
              tunnel: [_ w803] -> w789
              tunnel: [_ w802] -> w788
              tunnel: [_ w801] -> w791
              tunnel: [_ w800] -> w793
              tunnel: w792 -> [_ w799]
              tunnel: w787 -> [_ w798]
              tunnel: [_ w797] -> w785
              tunnel: [_ w796] -> w784
              tunnel: [_ w795] -> w783
              frame False {
              }
              frame True {
                n100 = case shown="True" w798 {
                  tunnel: [_ TRUE ("Enable Termination\nChar (T)")] -> w802
                  tunnel: [_ TRUE ("Connexion")] -> w804
                  tunnel: [_ TRUE ("Connexion Active")] -> w803
                  tunnel: w805 -> [_ w823]
                  tunnel: [_ w814] -> w801
                  tunnel: [_ "Connecté" ("Statut de connexion")] -> w800
                  tunnel: w799 -> [_ w809]
                  tunnel: [_ "Vitesse Max"] -> w797
                  tunnel: [_ TRUE ("EEPROM prête")] -> w796
                  tunnel: [_ w806] -> w795
                  frame False {
                  }
                  frame True {
                    n101 = Wait (ms)(milliseconds to wait=u32 100) -> ()  [unwired: 1 out]
                    n102 = Format Into String(format string="<CMD,PMAX:%d> ", error in=w823, "Poids Max") -> (resulting string=w806:string, error out=w825:errorcluster)  [unwired: 1 in]
                    n103 = Wait (ms)(milliseconds to wait=u32 100) -> ()  [unwired: 1 out]
                    n104 = VISA Write(VISA resource name=w809, write buffer=w806, error in (no error)=w825) -> (VISA resource name out=w817:refnum<visa-resource-name>, error out=w816:errorcluster)  [unwired: 1 out]
                    n105 = Format Into String(format string="<CMD,SPD:%d>", error in=w816, "Vitesse Max") -> (resulting string=w822:string, error out=w815:errorcluster)  [unwired: 1 in]
                    n106 = VISA Write(VISA resource name=w817, write buffer=w822, error in (no error)=w815) -> (error out=w814:errorcluster)  [unwired: 2 out]
                    n107 = One Button Dialog(message="Configuration envoyée au PIC !", button name ("OK")="OK") -> ()  [unwired: 1 out]
                  }
                }
              }
            }
          }
          frame True {
          }
        }
      }
      event "Ouverture Porte": Value Change {
        n108 = event-data() -> ()  [unwired: 1 in, 3 out]
        n109 = case shown="False" w844 {
          tunnel: w834 -> [w859 _]
          tunnel: w847 -> [w858 _]
          tunnel: w846 -> [w857 _]
          tunnel: [w856 _] -> w836
          tunnel: w845 -> [w855 _]
          tunnel: [w854 _] -> w843
          tunnel: [w853 _] -> w842
          tunnel: [w852 _] -> w841
          tunnel: [w851 _] -> w840
          tunnel: [w850 _] -> w839
          tunnel: [w849 _] -> w838
          tunnel: [w848 _] -> w837
          frame False {
            n110 = case shown="True" w855 {
              tunnel: w859 -> [_ w867]
              tunnel: w858 -> [_ w870]
              tunnel: w857 -> [_ w869]
              tunnel: [_ w868] -> w856
              tunnel: [_ w866] -> w854
              tunnel: [_ w865] -> w853
              tunnel: [_ w864] -> w852
              tunnel: [_ w863] -> w851
              tunnel: [_ w862] -> w850
              tunnel: [_ w861] -> w849
              tunnel: [_ w860] -> w848
              frame False {
              }
              frame True {
                n111 = case shown="True" w867 {
                  tunnel: w870 -> [_ w880]
                  tunnel: w869 -> [_ w879]
                  tunnel: [_ w878] -> w868
                  tunnel: [_ "Porte ouverte" ("Statut de connexion")] -> w866
                  tunnel: [_ TRUE ("Connexion")] -> w865
                  tunnel: [_ TRUE ("Connexion Active")] -> w864
                  tunnel: [_ TRUE ("Enable Termination\nChar (T)")] -> w863
                  tunnel: [_ TRUE ("Capteur IR")] -> w862
                  tunnel: [_ TRUE ("Cabine en mvt")] -> w861
                  tunnel: [_ w871] -> w860
                  frame False {
                  }
                  frame True {
                    w871 = "<CMD,DOOR:O>"
                    n112 = VISA Write(VISA resource name=w880, write buffer=w871, error in (no error)=w879) -> (error out=w878:errorcluster)  [unwired: 2 out]
                  }
                }
              }
            }
          }
          frame True {
          }
        }
      }
      event "Fermeture Porte": Value Change {
        n113 = event-data() -> ()  [unwired: 1 in, 3 out]
        n114 = case shown="False" w898 {
          tunnel: w901 -> [w914 _]
          tunnel: [w913 _] -> w887
          tunnel: w900 -> [w912 _]
          tunnel: w899 -> [w911 _]
          tunnel: w897 -> [w910 _]
          tunnel: [w909 _] -> w896
          tunnel: [w908 _] -> w894
          tunnel: [w907 _] -> w893
          tunnel: [w906 _] -> w892
          tunnel: [w905 _] -> w891
          tunnel: [w904 _] -> w890
          tunnel: [w903 _] -> w889
          tunnel: [w902 _] -> w888
          frame False {
            n115 = case shown="True" w911 {
              tunnel: w914 -> [_ w926]
              tunnel: [_ w925] -> w913
              tunnel: w912 -> [_ w924]
              tunnel: w910 -> [_ w923]
              tunnel: [_ w922] -> w909
              tunnel: [_ w921] -> w908
              tunnel: [_ w920] -> w907
              tunnel: [_ w919] -> w906
              tunnel: [_ w918] -> w905
              tunnel: [_ w917] -> w904
              tunnel: [_ w916] -> w903
              tunnel: [_ w915] -> w902
              frame False {
              }
              frame True {
                n116 = case shown="True" w924 {
                  tunnel: [_ w937] -> w925
                  tunnel: w926 -> [_ w936]
                  tunnel: w923 -> [_ w935]
                  tunnel: [_ TRUE ("Connexion")] -> w922
                  tunnel: [_ "Porte fermée" ("Statut de connexion")] -> w921
                  tunnel: [_ FALSE] -> w920
                  tunnel: [_ TRUE ("Connexion Active")] -> w919
                  tunnel: [_ TRUE ("Enable Termination\nChar (T)")] -> w918
                  tunnel: [_ TRUE ("Mode Manu")] -> w917
                  tunnel: [_ FALSE ("Capteur IR")] -> w916
                  tunnel: [_ w927] -> w915
                  frame False {
                  }
                  frame True {
                    w927 = "<CMD,DOOR:F>"
                    n117 = VISA Write(VISA resource name=w936, write buffer=w927, error in (no error)=w935) -> (error out=w937:errorcluster)  [unwired: 2 out]
                  }
                }
              }
            }
          }
          frame True {
          }
        }
      }
      event "Montée": Value Change {
        n118 = event-data() -> ()  [unwired: 1 in, 3 out]
        n119 = case shown="False" w957 {
          tunnel: [w969 _] -> w952
          tunnel: w956 -> [w968 _]
          tunnel: w955 -> [w967 _]
          tunnel: w954 -> [w966 _]
          tunnel: w951 -> [w965 _]
          tunnel: [w964 _] -> w950
          tunnel: [w963 _] -> w949
          tunnel: [w962 _] -> w948
          tunnel: [w961 _] -> w947
          tunnel: [w960 _] -> w946
          tunnel: [w959 _] -> w945
          tunnel: [w958 _] -> w944
          frame False {
            n120 = case shown="True" w968 {
              tunnel: [_ w980] -> w969
              tunnel: w967 -> [_ w979]
              tunnel: w966 -> [_ w978]
              tunnel: w965 -> [_ w977]
              tunnel: [_ w976] -> w964
              tunnel: [_ w975] -> w963
              tunnel: [_ w974] -> w962
              tunnel: [_ w973] -> w961
              tunnel: [_ w972] -> w960
              tunnel: [_ w971] -> w959
              tunnel: [_ w970] -> w958
              frame False {
              }
              frame True {
                n121 = case shown="True" w979 {
                  tunnel: [_ w990] -> w980
                  tunnel: w978 -> [_ w989]
                  tunnel: w977 -> [_ w988]
                  tunnel: [_ TRUE ("EEPROM prête")] -> w976
                  tunnel: [_ TRUE ("Connexion Active")] -> w975
                  tunnel: [_ "Montée activée" ("Statut de connexion")] -> w974
                  tunnel: [_ TRUE ("Cabine en mvt")] -> w973
                  tunnel: [_ TRUE ("Connexion")] -> w972
                  tunnel: [_ w982] -> w971
                  tunnel: [_ TRUE ("Mode Manu")] -> w970
                  frame False {
                  }
                  frame True {
                    w982 = "<CMD,MOT:UP> "
                    n122 = VISA Write(VISA resource name=w989, write buffer=w982, error in (no error)=w988) -> (error out=w990:errorcluster)  [unwired: 2 out]
                  }
                }
              }
            }
          }
          frame True {
          }
        }
      }
      event "Descente": Value Change {
        n123 = event-data() -> ()  [unwired: 1 in, 3 out]
        n124 = case shown="False" w1007 {
          tunnel: [w1022 _] -> w1005
          tunnel: w1010 -> [w1021 _]
          tunnel: w1009 -> [w1020 _]
          tunnel: w1008 -> [w1019 _]
          tunnel: w1004 -> [w1018 _]
          tunnel: [w1017 _] -> w1003
          tunnel: [w1016 _] -> w1002
          tunnel: [w1015 _] -> w1001
          tunnel: [w1014 _] -> w1000
          tunnel: [w1013 _] -> w999
          tunnel: [w1012 _] -> w998
          tunnel: [w1011 _] -> w997
          frame False {
            n125 = case shown="True" w1019 {
              tunnel: [_ w1033] -> w1022
              tunnel: w1021 -> [_ w1032]
              tunnel: w1020 -> [_ w1031]
              tunnel: w1018 -> [_ w1030]
              tunnel: [_ w1029] -> w1017
              tunnel: [_ w1028] -> w1016
              tunnel: [_ w1027] -> w1015
              tunnel: [_ w1026] -> w1014
              tunnel: [_ w1025] -> w1013
              tunnel: [_ w1024] -> w1012
              tunnel: [_ w1023] -> w1011
              frame False {
              }
              frame True {
                n126 = case shown="True" w1031 {
                  tunnel: [_ w1043] -> w1033
                  tunnel: w1032 -> [_ w1042]
                  tunnel: w1030 -> [_ w1041]
                  tunnel: [_ TRUE ("Connexion")] -> w1029
                  tunnel: [_ TRUE ("Connexion Active")] -> w1028
                  tunnel: [_ TRUE ("Enable Termination\nChar (T)")] -> w1027
                  tunnel: [_ TRUE ("Cabine en mvt")] -> w1026
                  tunnel: [_ TRUE ("Mode Manu")] -> w1025
                  tunnel: [_ w1035] -> w1024
                  tunnel: [_ "Descente activée" ("Statut de connexion")] -> w1023
                  frame False {
                  }
                  frame True {
                    w1035 = "<CMD,MOT:DWN>"
                    n127 = VISA Write(VISA resource name=w1042, write buffer=w1035, error in (no error)=w1041) -> (error out=w1043:errorcluster)  [unwired: 2 out]
                  }
                }
              }
            }
          }
          frame True {
          }
        }
      }
      event "Stop": Value Change {
        n128 = event-data() -> ()  [unwired: 1 in, 3 out]
        n129 = case shown="True" w1055 {
          tunnel: w1058 -> [_ w1067]
          tunnel: w1057 -> [_ w1066]
          tunnel: [_ w1065] -> w1056
          tunnel: [_ "Acquisition arrêtée " ("Statut de connexion")] -> w1044
          tunnel: [_ w1063] -> w1054
          tunnel: [_ TRUE ("Connexion")] -> w1053
          tunnel: [_ TRUE ("Connexion Active")] -> w1052
          tunnel: [_ TRUE ("Enable Termination\nChar (T)")] -> w1051
          frame False {
          }
          frame True {
            w1063 = "<CMD,PAUSE>" ("write buffer")
            n130 = VISA Write(VISA resource name=w1067, write buffer=w1063, error in (no error)=w1066) -> (error out=w1065:errorcluster)  [unwired: 2 out]
          }
        }
      }
      event "Start": Value Change {
        n131 = event-data() -> ()  [unwired: 1 in, 3 out]
        n132 = case shown="False" w1075 {
          tunnel: w1082 -> [w1092 _]
          tunnel: w1081 -> [w1091 _]
          tunnel: [w1090 _] -> w1080
          tunnel: [w1089 _] -> w1079
          tunnel: [w1088 _] -> w1078
          tunnel: [w1087 _] -> w1077
          tunnel: w1076 -> [w1086 _]
          tunnel: [w1085 _] -> w1074
          tunnel: [w1084 _] -> w1073
          frame False {
            n133 = case shown="True" w1086 {
              tunnel: w1092 -> [_ w1100]
              tunnel: w1091 -> [_ w1099]
              tunnel: [_ w1098] -> w1090
              tunnel: [_ "Système démarré" ("Statut de connexion")] -> w1085
              tunnel: [_ TRUE ("Connexion")] -> w1089
              tunnel: [_ TRUE ("Connexion Active")] -> w1088
              tunnel: [_ TRUE ("Enable Termination\nChar (T)")] -> w1087
              tunnel: [_ w1093] -> w1084
              frame False {
              }
              frame True {
                w1093 = "<CMD,START> " ("write buffer")
                n134 = VISA Write(VISA resource name=w1100, write buffer=w1093, error in (no error)=w1099) -> (error out=w1098:errorcluster)  [unwired: 2 out]
              }
            }
          }
          frame True {
          }
        }
      }
      event "Clear": Value Change {
        n135 = event-data() -> ()  [unwired: 1 in, 3 out]
        n136 = case shown="True" w1107 {
          tunnel: [_ w1121] -> w1113
          tunnel: w1114 -> [_ w1121]
          tunnel: [_ string[][] [] ("Table Control")] -> w1112
          tunnel: [_ "Connecté" ("Statut de connexion")] -> w1111
          tunnel: [_ TRUE ("Connexion")] -> w1110
          tunnel: [_ TRUE ("Connexion Active")] -> w1109
          tunnel: [_ TRUE ("Enable Termination\nChar (T)")] -> w1108
          frame False {
          }
          frame True {
          }
        }
      }
      event "Sauvegarder": Value Change {
        n137 = event-data() -> ()  [unwired: 1 in, 3 out]
        n138 = case shown="True" w1122 {
          tunnel: w1136 -> [_ w1144]
          tunnel: [_ w1144] -> w1135
          tunnel: [_ TRUE ("Connexion")] -> w1133
          tunnel: [_ TRUE ("Enable Termination\nChar (T)")] -> w1132
          tunnel: [_ TRUE ("Connexion Active")] -> w1131
          tunnel: [_ "Fichier sauvegardé" ("Statut de connexion")] -> w1130
          frame False {
          }
          frame True {
            n139 = call "Sauvegarde.vi"("Table Control"=w1144) -> ()  [unwired: 11 in]
            n140 = One Button Dialog(message="Fichier sauvegardé avec succès !", button name ("OK")="OK") -> ()  [unwired: 1 out]
          }
        }
      }
      event "Clear RX": Value Change {
        n141 = event-data() -> ()  [unwired: 1 in, 3 out]
        n142 = case shown="True" w1155 {
          tunnel: [_ TRUE ("Enable Termination\nChar (T)")] -> w1159
          tunnel: [_ TRUE ("Connexion")] -> w1160
          tunnel: [_ "" ("Trames Recues")] -> w1161
          tunnel: [_ w1164] -> w1157
          tunnel: w1158 -> [_ w1164]
          tunnel: [_ TRUE ("Connexion Active")] -> w1156
          tunnel: [_ "Trames reçues effacées" ("Statut de connexion")] -> w1154
          frame False {
          }
          frame True {
          }
        }
      }
      event "Clear TX": Value Change {
        n143 = event-data() -> ()  [unwired: 1 in, 3 out]
        n144 = case shown="True" w1179 {
          tunnel: [_ TRUE ("Enable Termination\nChar (T)")] -> w1181
          tunnel: [_ TRUE ("Connexion")] -> w1183
          tunnel: [_ "" ("Trames Recues")] -> w1180
          tunnel: [_ TRUE ("Connexion Active")] -> w1182
          tunnel: [_ w1185] -> w1177
          tunnel: w1178 -> [_ w1185]
          tunnel: [_ "Trames envoyées effacées" ("Statut de connexion")] -> w1176
          frame False {
          }
          frame True {
          }
        }
      }
    }
    "Etage Actuel" <- w25
    "Nb trajet" <- w7
    "Graphique 1 Position en fonction du temps" <- w22
    "Graphique 2 Poids en fonction du temps" <- w13
    "Connexion Active" <- w44
    "Porte Ouverte" <- w37
    "Surcharge" <- w33
    "Alarme" <- w36
    "Arrêt urgence" <- w38
    "Mode Auto" <- w40
    "Mode Manu" <- w41
    "Cabine en mvt" <- w39
    "EEPROM prête" <- w34
    "Capteur IR" <- w42
    "Connexion" <- w47
    "Statut de connexion" <- w43
    "Trajets total" <- w8
    "Dernier étage" <- w35
    "Trames Recues" <- w17
    "LCD" <- w20
    "Table Control" <- w28
    "Trames envoyés" <- w23
    "Direction" <- w19
    "Poids cabine" <- w21
    "Vitesse sauvegarder" <- w27
    "Vitesse Moteur" <- w26
    n145 = call <vilib>:"Simple Error Handler.vi"("error in (no error)"=w51) -> ()  [unwired: 4 in, 5 out]
  }
